vi "zdotc - Dot Product with Conjugation (CDB).vi"(5 "yInc":i32=1, 7 "xInc":i32=1, 10 "y":cdb[](array[numeric]), 11 "x":cdb[](array[numeric])) -> (0 "error":i32, 3 "zdotc":cdb)   [LabVIEW 2020, in "NI_AALBLAS.lvlib"]
doc: "Calculates the conjugated dot product of two complex vectors."
uses:
  NI_AALBLAS.lvlib
  Fucntion.ctl
  BLAS1 Utility(CDB).vi
panel:
  # "zdotc=conjg(x')*y"
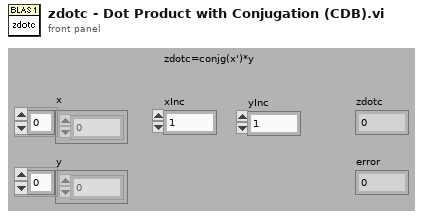
[diagram p1: front panel]
types:
  T1 = typedef "NI_AALBLAS.lvlib/fucntion.ctl" = u16
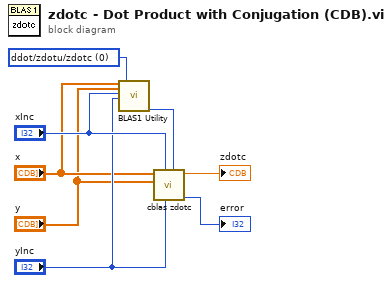
[diagram p0: block diagram]
diagram:
  w1 = T1 0 items=["ddot/zdotu/zdotc", "daxpy/zaxpy", "dnrm2/dznrm2", "dasum/dzasum", "dcopy/zcopy", "dswap/zswap", "drotm", "drot/zdrot", "idamax/izamax", "idamin/izamin", "dgemv/zgemv", "dsymv/zhemv", "dtrmv/ztrmv", "dsyr/zher", "dsyr2/zher2", "dger/zgeru/zgerc", "dtrsv/ztrsv", "dgemm/zgemm", "dsymm/zsymm/zhemm", "dtrmm/ztrmm", "dsyrk/zsyrk/zherk", "dsyr2k/zsyr2k/zher2k", "dtrsm/ztrsm"] ("function")
  n1 = call-poly "BLAS1 Utility.vi"("x"="x", "y"="y", "xInc"="xInc", "yInc"="yInc", "function"=w1) -> ("n"=w2:i32)  [unwired: 14 out]
  n2 = call "cblas zdotc.vi"("n"=w2, "incy"="yInc", "incx"="xInc", "y"="y", "x"="x") -> ("error"=→"error":i32, "zdotc"=→"zdotc":cdb)  [unwired: 5 out]
